vi "Change value.vi"(9 "Task name":string, 10 "Data string":string, 11 "DAQmx Tasks":T1(array[cluster])) -> (3 "tableau en sortie":T1(array[cluster]))   [LabVIEW 2015, in "DAQmxTaskContainer.lvclass"]
uses:
  DAQmxTaskContainer.lvclass
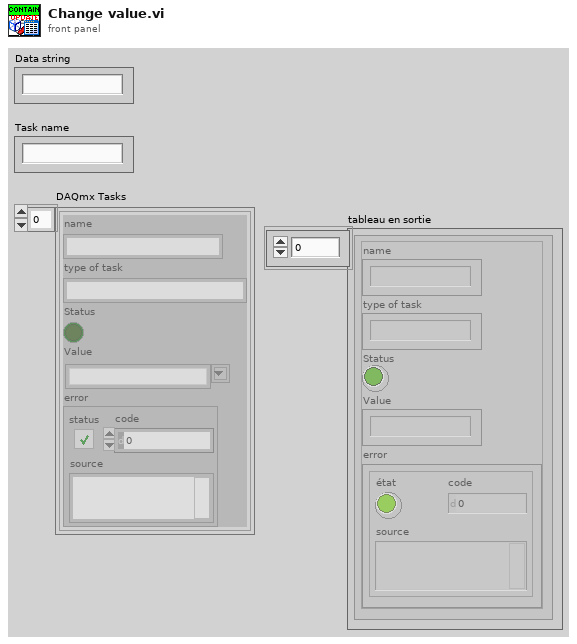
[diagram p1: front panel]
types:
  T1 = cluster{"name":string, "type of task":string, "Status":bool, "Value":string, "error":errorcluster}[]
  T2 = cluster{"name":string, "type of task":string, "Status":bool, "Value":string, "error":errorcluster}
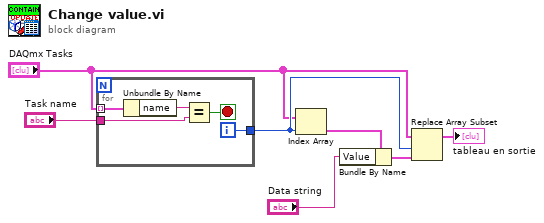
[diagram p0: block diagram]
diagram:
  n1 = for {
    tunnel: "DAQmx Tasks" -> [w12] mode=indexing
    tunnel: "Task name" -> [w10]
    tunnel: [w8] -> w5
    i -> [w8]
    stop <- w9 stop-if-true
    n2 = Unbundle By Name(w12) -> ("name"=w11:string)
    n3 = Equal?(x=w11, y=w10) -> (x = y?=w9:bool)
  }
  n4 = Index Array(array="DAQmx Tasks", index=w5) -> (element=w3:T2)
  n5 = Bundle By Name(cluster=w3, "Value"="Data string") -> (w6:T2)
  n6 = Replace Array Subset(array="DAQmx Tasks", new element=w6, index=w5) -> (→"tableau en sortie":T1)
